vi "BuildPageArray.vi"(8 "error in (no error)":errorcluster, 10 "Config File Path":path) -> (0 "error out":errorcluster, 2 "Num Pages":i32, 3 "Array":refnum<class "Slide.lvclass">[](array[class]))   [LabVIEW 2017]
uses:
  Presentation/Slide/Slide.lvclass
  Presentation/Slide/SlideType.ctl
  <vilib>/regexp/Match Regular Expression.xnode
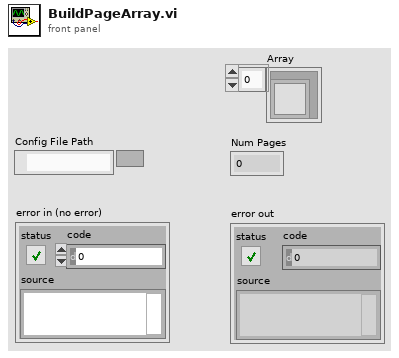
[diagram p1: front panel]
types:
  T1 = typedef "Slide.lvclass/SlideType.ctl" = enum16{"Image", "FP", "BD", "VI-Run"}
  T2 = cluster{i32, "BD Slide":refnum<class "Slide.lvclass">}
  T3 = cluster{i32, "BD Slide":refnum<class "Slide.lvclass">}[]
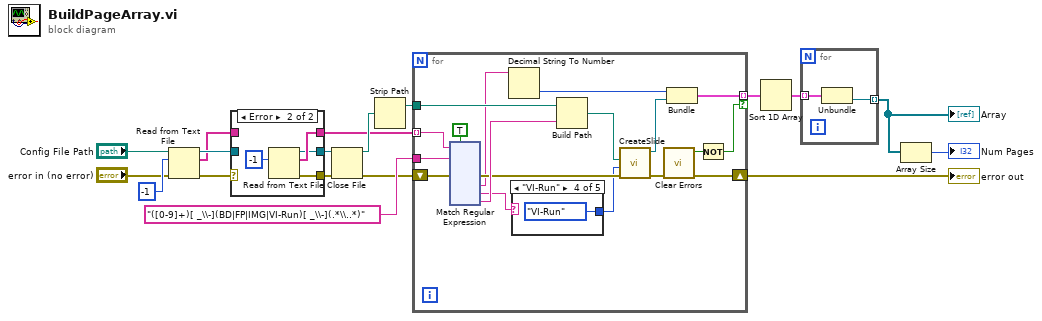
[diagram p0: block diagram]
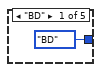
[diagram p3: hidden frame]
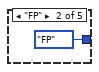
[diagram p4: hidden frame]
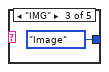
[diagram p5: hidden frame]
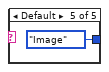
[diagram p6: hidden frame]
diagram:
  n1 = Read from Text File(file (use dialog)="Config File Path", count=-1, error in="error in (no error)") -> (refnum out=w15:refnum<file>, text=w4:string[], error out=w5:errorcluster)  [unwired: 1 in, 1 out]
  n2 = case shown="Error" w5 {
    selector: w5 -> [w21 _]
    tunnel: w15 -> [w19 _]
    tunnel: [w21 w25] -> w14
    tunnel: [w20 w23] -> w3
    tunnel: w4 -> [w20 _]
    tunnel: [w19 w22] -> w1
    frame No Error {
    }
    frame Error {
      n3 = Read from Text File(count=-1) -> (refnum out=w22:refnum<file>, text=w23:string[], error out=w25:errorcluster)  [unwired: 3 in, 1 out]
    }
  }
  n4 = Close File(refnum=w1, error in=w14) -> (path=w18:path, error out=w2:errorcluster)
  n5 = Strip Path(path=w18) -> (stripped path=w11:path)  [unwired: 1 out]
  n6 = for {
    tunnel: w3 -> [w42] mode=indexing
    shift-right: [w28] -> w9
    shift-left: w2 -> [w40]
    tunnel: "([0-9]+)[ _\\-](BD|FP|IMG|VI-Run)[ _\\-](.*\\..*)" -> [w39]
    tunnel: w11 -> [w38]
    tunnel: [w29] -> w8 mode=indexing if=w26
    n7 = xnode "Match Regular Expression"("input string"=w42, "regular expression"=w39, "error in"=w40, "ignore case? (F)"=TRUE) -> ("error out"=w36:errorcluster, "submatch 1"=w32:string, "submatch 2"=w37:string, "submatch 3"=w43:string)  [unwired: 2 in, 4 out]
    n8 = Decimal String To Number(string=w32) -> (number=w31:i32)  [unwired: 2 in, 1 out]
    n9 = case shown="\"VI-Run\"" w37 {
      tunnel: [SlideType."BD" ("Type") SlideType."FP" ("Type") SlideType."Image" ("Type") SlideType."VI-Run" ("Type") SlideType."Image" ("Type")] -> w34
      frame "BD" {
      }
      frame "FP" {
      }
      frame "IMG" {
      }
      frame "VI-Run" {
      }
      frame Default {
      }
    }
    n10 = Build Path(base path=w38, name or relative path=w43) -> (appended path=w33:path)
    n11 = call "CreateSlide.vi"("error in (no error)"=w36, "Type (FP)"=w34, "Path"=w33) -> ("error out"=w35:errorcluster, "BD Slide"=w30:refnum<class "Slide.lvclass">)  [unwired: 7 in]
    n12 = call <vilib>:"Clear Errors.vi"("error in (no error)"=w35) -> ("error out"=w28:errorcluster, "specific error cleared?"=w27:bool)  [unwired: 5 in]
    n13 = Bundle(w31, "BD Slide"=w30) -> (w29:T2)  [unwired: 1 in]
    n14 = Not(x=w27) -> (.not. x?=w26:bool)
  }
  "error out" <- w9
  n15 = Sort 1D Array(array=w8) -> (sorted array=w7:T3)
  n16 = for {
    tunnel: w7 -> [w168] mode=indexing
    tunnel: [w167] -> w6 mode=indexing
    n17 = Unbundle(w168) -> ("BD Slide"=w167:refnum<class "Slide.lvclass">)  [unwired: 1 out]
  }
  "Array" <- w6
  n18 = Array Size(array=w6) -> (size(s)=→"Num Pages":i32)
